vi "Get MetaData from Configurations.vi"(8 "error in":errorcluster, 10 "measurement plugin service in":refnum<class "Measurement Plugin Service.lvclass">, 11 "configuration cluster":variant) -> (0 "error out":errorcluster, 2 "measurement plugin service out":refnum<class "Measurement Plugin Service.lvclass">, 3 "configuration parameters":T1[](array[typedef]))   [LabVIEW 2021, in "NI Measurement Plug-In SDK.lvlib"]
uses:
  NI Measurement Plug-In SDK.lvlib
  TypeDefs/Configuration Parameter.ctl
  TypeDefs/Parameter Annotations Entry.ctl
  Measurement Plugin Service/Measurement Plugin Service.lvclass
  <vilib>/Utility/Data Type/NI_Data Type.lvlib
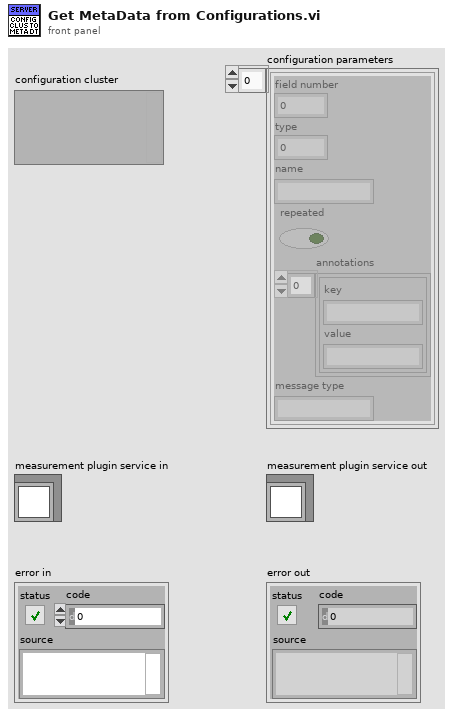
[diagram p1: front panel]
types:
  T1 = typedef "NI Measurement Plug-In SDK.lvlib/Configuration Parameter.ctl" = cluster{"field number":i32, "type":i32, "name":string, "repeated":bool, "annotations":T2[], "message type":string}
  T2 = typedef "NI Measurement Plug-In SDK.lvlib/Parameter Annotations Entry.ctl" = cluster{"key":string, "value":string}
  T3 = typedef "NI Measurement Plug-In SDK.lvlib/Measurement Plugin Service.lvclass/Plugin Paths.ctl" = cluster{"get service descriptor VI path":path, "get type specializations VI path":path, "get UI details VI path":path, "measurement logic VI path":path, "measurement configuration ctl path":path, "measurement results ctl path":path}
  T4 = cluster{"Parameter Name":string, "Annotations":T2[]}[]
  T5 = typedef "NI Measurement Plug-In SDK.lvlib/Google Protobuf Field Kind.ctl" = enum32{"TYPE_UNKNOWN", "TYPE_DOUBLE", "TYPE_FLOAT", "TYPE_INT64", "TYPE_UINT64", "TYPE_INT32", "TYPE_FIXED64", "TYPE_FIXED32", "TYPE_BOOL", "TYPE_STRING", "TYPE_GROUP", "TYPE_MESSAGE", "TYPE_BYTES", "TYPE_UINT32", "TYPE_ENUM", "TYPE_SFIXED32", "TYPE_SFIXED64", "TYPE_SINT32", "TYPE_SINT64"}
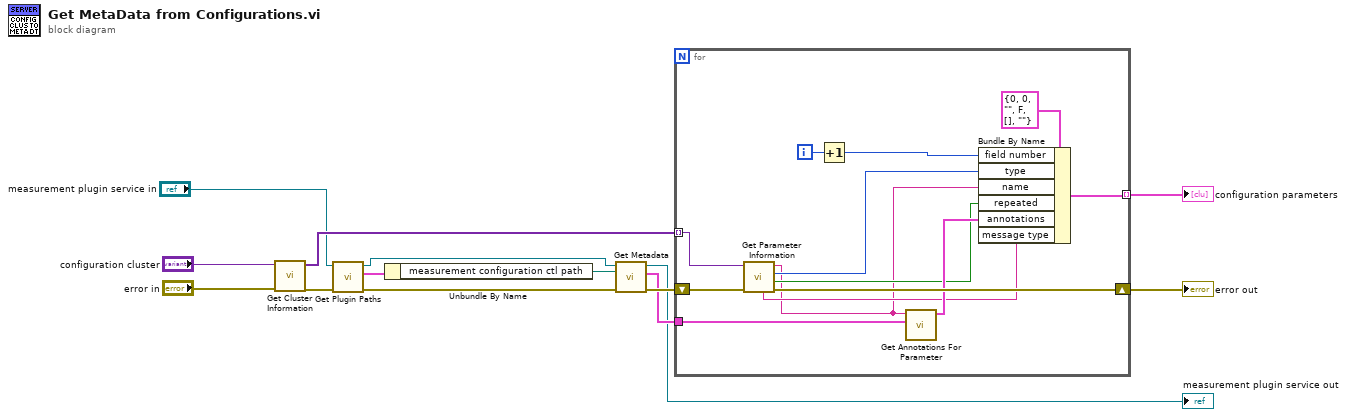
[diagram p0: block diagram]
diagram:
  n1 = call <vilib>:"Get Cluster Information.vi"("error in (no error)"="error in", "variant"="configuration cluster") -> ("error out"=w7:errorcluster, "cluster elements"=w14:variant[])  [unwired: 8 in]
  n2 = call-dynamic "Get Plugin Paths.vi"("error in"=w7, "measurement plugin service in"="measurement plugin service in") -> ("error out"=w10:errorcluster, "plugin paths"=w11:T3, "measurement plugin service out"=w9:refnum<class "Measurement Plugin Service.lvclass">)  [unwired: 7 in]
  n3 = Unbundle By Name(w11) -> ("measurement configuration ctl path"=w12:path)
  n4 = call "Get Metadata.vi"("error in"=w10, "measurement control path"=w12, "measurement plugin service in"=w9) -> ("error out"=w8:errorcluster, "metadata value"=w5:T4, "measurement plugin service out"=→"measurement plugin service out":refnum<class "Measurement Plugin Service.lvclass">)  [unwired: 5 in]
  n5 = for {
    tunnel: w14 -> [w21] mode=indexing
    tunnel: [w20] -> w2 mode=indexing
    shift-right: [w25] -> w3
    shift-left: w8 -> [w22]
    tunnel: w5 -> [w23]
    i -> [w27]
    n6 = call "Get Parameter Information.vi"("error in"=w22, "variant data"=w21) -> ("error out"=w25:errorcluster, "repeated"=w16:bool, "grpc type"=w17:T5, "name"=w15:string, "message type"=w18:string)  [unwired: 5 in]
    n7 = Increment(x=w27) -> (x+1=w26:i32)
    n8 = call "Get Annotations For Parameter.vi"("metadata value"=w23, "parameter name"=w15) -> ("annotations"=w24:T2[])  [unwired: 9 in]
    n9 = Bundle By Name(cluster=T1 {"field number"=0, "type"=0, "name"="", "repeated"=FALSE, "annotations"=[], "message type"=""} ("ConfigurationParameter"), "field number"=w26, "type"=w17, "name"=w15, "repeated"=w16, "annotations"=w24, "message type"=w18) -> (w20:T1)
  }
  "error out" <- w3
  "configuration parameters" <- w2
